vi "UIinit_Main.vi"(10 "VIref":refnum<vi>, 11 "Language":refnum<vi>) -> ()   [LabVIEW 2015]
uses:
  GlobalVar.vi
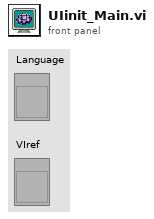
[diagram p1: front panel]
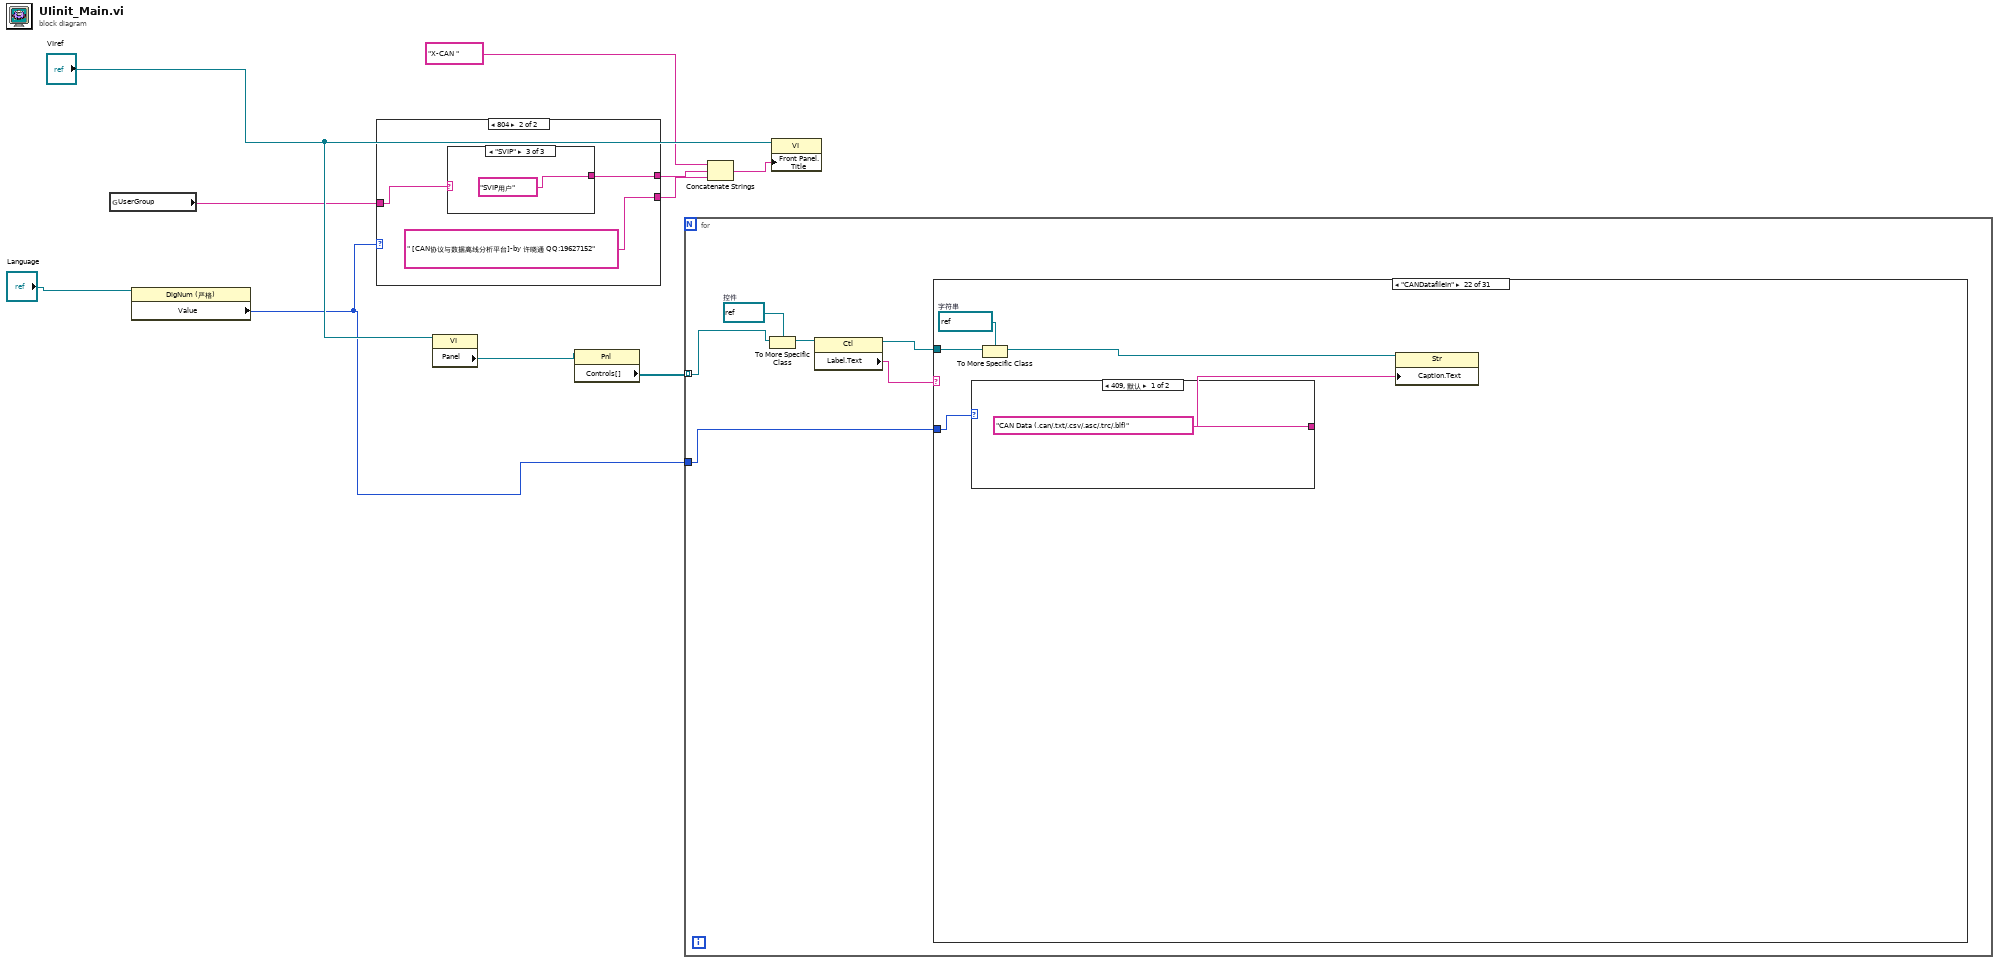
[diagram p0: block diagram]
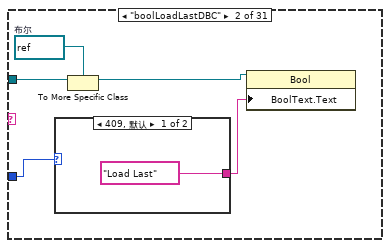
[diagram p3: hidden frame]
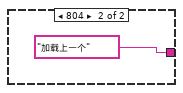
[diagram p4: hidden frame]
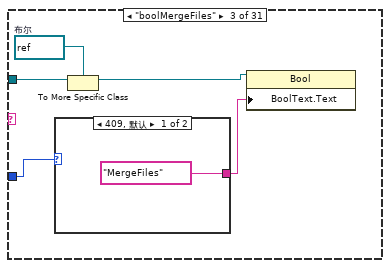
[diagram p5: hidden frame]
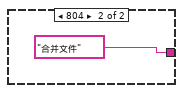
[diagram p6: hidden frame]
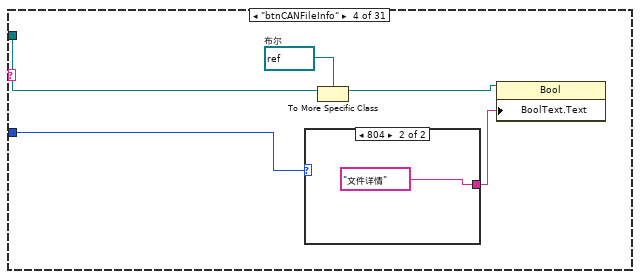
[diagram p7: hidden frame]
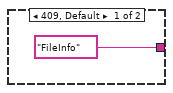
[diagram p8: hidden frame]
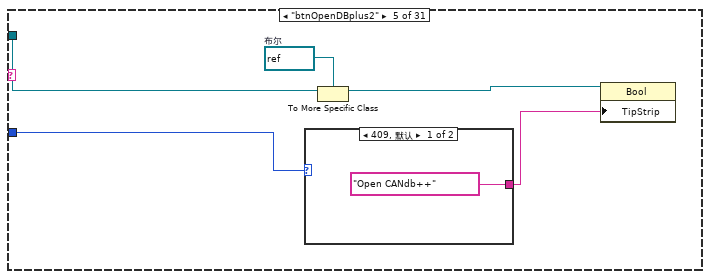
[diagram p9: hidden frame]
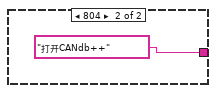
[diagram p10: hidden frame]
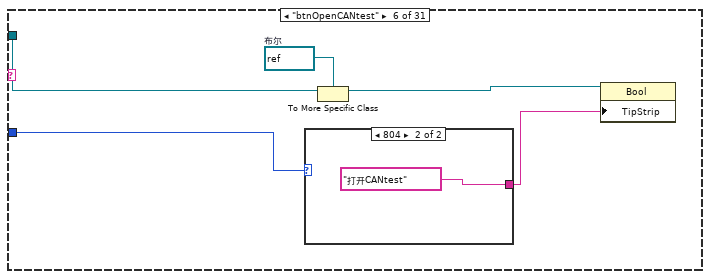
[diagram p11: hidden frame]
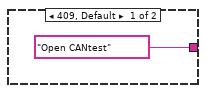
[diagram p12: hidden frame]
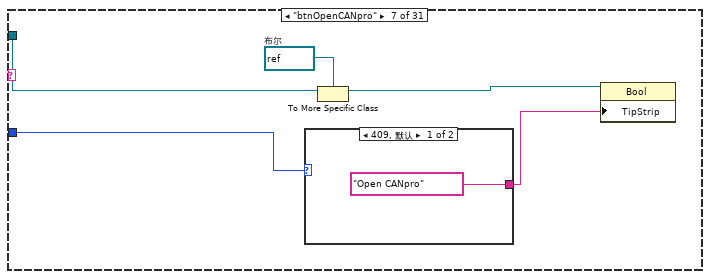
[diagram p13: hidden frame]
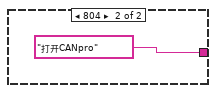
[diagram p14: hidden frame]
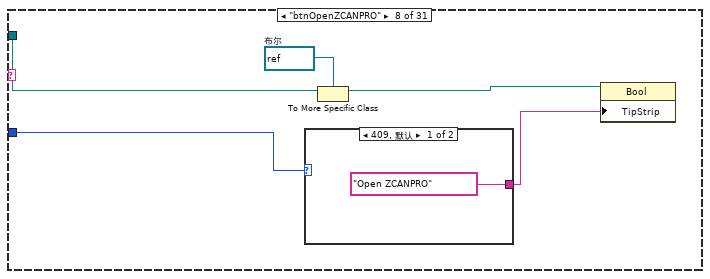
[diagram p15: hidden frame]
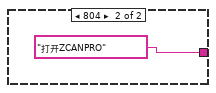
[diagram p16: hidden frame]
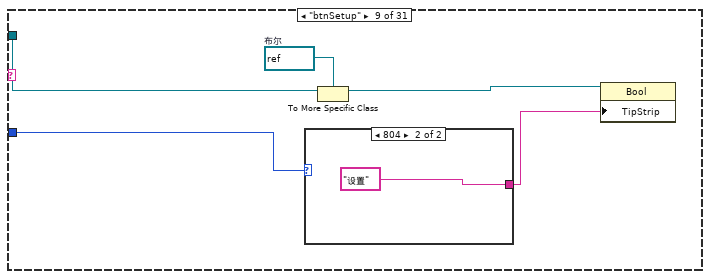
[diagram p17: hidden frame]
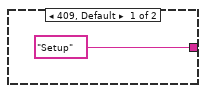
[diagram p18: hidden frame]
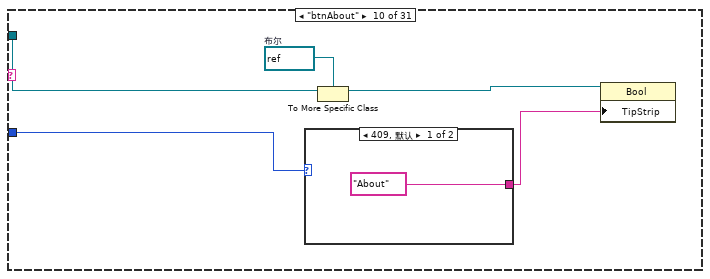
[diagram p19: hidden frame]
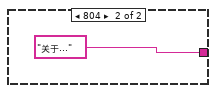
[diagram p20: hidden frame]
diagram:
  n1 = global read "GlobalVar.vi" "UserGroup"() -> (w2:string)
  n2 = property class="DigNum (严格)"(reference="Language") -> ("Value"=w6:u32)  [unwired: 1 in, 2 out]
  n3 = case shown="804" w6 {
    tunnel: [w12 " [CAN协议与数据离线分析平台]-by 许晓通 QQ:19627152"] -> w5
    tunnel: [w11 w13] -> w4
    tunnel: w2 -> [w11 w14]
    frame 409, Default {
      w12 = " [CAN Offline Analysis Platform]-by Jay Sur E-mail:jaysur@foxmail.com"  # [CAN Offline Analysis Platform]-by Jay Sur E-mail:jaysur@foxmail.com
    }
    frame 804 {
      n4 = case shown="\"SVIP\"" w14 {
        tunnel: ["普通用户" "VIP用户" "SVIP用户"] -> w13
        frame "假", Default {
        }
        frame "VIP" {
        }
        frame "SVIP" {
        }
      }
    }
  }
  n5 = property class="VI"(reference="VIref") -> ("Panel"=w7:refnum<vi>)  [unwired: 1 in, 2 out]
  n6 = property class="Pnl"(reference=w7) -> ("Controls[]"=w8:refnum<vi>[])  [unwired: 1 in, 2 out]
  n7 = for {
    tunnel: w8 -> [w19] mode=indexing
    tunnel: w6 -> [w20]
    w24 = refnum<vi> refnum  # 控件
    n8 = To More Specific Class(target class=w24, reference=w19) -> (specific class reference=w23:refnum<vi>)  [unwired: 1 in, 1 out]
    n9 = property class="Ctl"(reference=w23) -> (reference out=w21:refnum<vi>, "Label.Text"=w22:string)  [unwired: 1 in, 1 out]
    n10 = case shown="\"CANDatafileIn\"" w22 {
      tunnel: w21 -> [_ w28 w35 w42 w49 w56 w63 w70 w77 w84 w91 w98 w105 w113 w123 w132 w139 w146 w153 w160 w167 w174 w181 w188 w195 w202 w209 w216 w223 w231 w287]
      tunnel: w20 -> [_ w29 w36 w43 w50 w57 w64 w71 w78 w85 w92 w99 w106 w114 w124 w133 w140 w147 w154 w161 w168 w175 w182 w189 w196 w203 w210 w217 w224 w227 w292]
      frame "假", Default {
      }
      frame "boolLoadLastDBC" {
        w27 = refnum<vi> refnum  # 布尔
        n11 = case shown="409, 默认" w29 {
          tunnel: ["Load Last" "加载上一个"] -> w25
          frame 409, Default {
          }
          frame 804 {
          }
        }
        n12 = To More Specific Class(target class=w27, reference=w28) -> (specific class reference=w26:refnum<vi>)  [unwired: 1 in, 1 out]
        n13 = property class="Bool"(reference=w26, "BoolText.Text"=w25) -> ()  [unwired: 1 in, 2 out]
      }
      frame "boolMergeFiles" {
        w34 = refnum<vi> refnum  # 布尔
        n14 = case shown="409, 默认" w36 {
          tunnel: ["MergeFiles" "合并文件"] -> w32
          frame 409, Default {
          }
          frame 804 {
          }
        }
        n15 = To More Specific Class(target class=w34, reference=w35) -> (specific class reference=w33:refnum<vi>)  [unwired: 1 in, 1 out]
        n16 = property class="Bool"(reference=w33, "BoolText.Text"=w32) -> ()  [unwired: 1 in, 2 out]
      }
      frame "btnCANFileInfo" {
        w41 = refnum<vi> refnum  # 布尔
        n17 = case shown="804" w43 {
          tunnel: ["FileInfo" "文件详情"] -> w39
          frame 409, Default {
          }
          frame 804 {
          }
        }
        n18 = To More Specific Class(target class=w41, reference=w42) -> (specific class reference=w40:refnum<vi>)  [unwired: 1 in, 1 out]
        n19 = property class="Bool"(reference=w40, "BoolText.Text"=w39) -> ()  [unwired: 1 in, 2 out]
      }
      frame "btnOpenDBplus2" {
        w48 = refnum<vi> refnum  # 布尔
        n20 = case shown="409, 默认" w50 {
          tunnel: ["Open CANdb++" "打开CANdb++"] -> w46
          frame 409, Default {
          }
          frame 804 {
          }
        }
        n21 = To More Specific Class(target class=w48, reference=w49) -> (specific class reference=w47:refnum<vi>)  [unwired: 1 in, 1 out]
        n22 = property class="Bool"(reference=w47, "TipStrip"=w46) -> ()  [unwired: 1 in, 2 out]
      }
      frame "btnOpenCANtest" {
        w55 = refnum<vi> refnum  # 布尔
        n23 = case shown="804" w57 {
          tunnel: ["Open CANtest" "打开CANtest"] -> w53
          frame 409, Default {
          }
          frame 804 {
          }
        }
        n24 = To More Specific Class(target class=w55, reference=w56) -> (specific class reference=w54:refnum<vi>)  [unwired: 1 in, 1 out]
        n25 = property class="Bool"(reference=w54, "TipStrip"=w53) -> ()  [unwired: 1 in, 2 out]
      }
      frame "btnOpenCANpro" {
        w62 = refnum<vi> refnum  # 布尔
        n26 = case shown="409, 默认" w64 {
          tunnel: ["Open CANpro" "打开CANpro"] -> w60
          frame 409, Default {
          }
          frame 804 {
          }
        }
        n27 = To More Specific Class(target class=w62, reference=w63) -> (specific class reference=w61:refnum<vi>)  [unwired: 1 in, 1 out]
        n28 = property class="Bool"(reference=w61, "TipStrip"=w60) -> ()  [unwired: 1 in, 2 out]
      }
      frame "btnOpenZCANPRO" {
        w69 = refnum<vi> refnum  # 布尔
        n29 = case shown="409, 默认" w71 {
          tunnel: ["Open ZCANPRO" "打开ZCANPRO"] -> w67
          frame 409, Default {
          }
          frame 804 {
          }
        }
        n30 = To More Specific Class(target class=w69, reference=w70) -> (specific class reference=w68:refnum<vi>)  [unwired: 1 in, 1 out]
        n31 = property class="Bool"(reference=w68, "TipStrip"=w67) -> ()  [unwired: 1 in, 2 out]
      }
      frame "btnSetup" {
        w76 = refnum<vi> refnum  # 布尔
        n32 = case shown="804" w78 {
          tunnel: ["Setup" "设置"] -> w74
          frame 409, Default {
          }
          frame 804 {
          }
        }
        n33 = To More Specific Class(target class=w76, reference=w77) -> (specific class reference=w75:refnum<vi>)  [unwired: 1 in, 1 out]
        n34 = property class="Bool"(reference=w75, "TipStrip"=w74) -> ()  [unwired: 1 in, 2 out]
      }
      frame "btnAbout" {
        w83 = refnum<vi> refnum  # 布尔
        n35 = case shown="409, 默认" w85 {
          tunnel: ["About" "关于..."] -> w81
          frame 409, Default {
          }
          frame 804 {
          }
        }
        n36 = To More Specific Class(target class=w83, reference=w84) -> (specific class reference=w82:refnum<vi>)  [unwired: 1 in, 1 out]
        n37 = property class="Bool"(reference=w82, "TipStrip"=w81) -> ()  [unwired: 1 in, 2 out]
      }
      frame "btnDonate" {
        w90 = refnum<vi> refnum  # 布尔
        n38 = case shown="804" w92 {
          tunnel: ["Donate" "捐赠"] -> w88
          frame 409, Default {
          }
          frame 804 {
          }
        }
        n39 = To More Specific Class(target class=w90, reference=w91) -> (specific class reference=w89:refnum<vi>)  [unwired: 1 in, 1 out]
        n40 = property class="Bool"(reference=w89, "TipStrip"=w88) -> ()  [unwired: 1 in, 2 out]
      }
      frame "btnUpdateChk" {
        w97 = refnum<vi> refnum  # 布尔
        n41 = case shown="409, 默认" w99 {
          tunnel: ["Check Upadte" "检查更新"] -> w95
          frame 409, Default {
          }
          frame 804 {
          }
        }
        n42 = To More Specific Class(target class=w97, reference=w98) -> (specific class reference=w96:refnum<vi>)  [unwired: 1 in, 1 out]
        n43 = property class="Bool"(reference=w96, "TipStrip"=w95) -> ()  [unwired: 1 in, 2 out]
      }
      frame "ClearSelectedSig" {
        w104 = refnum<vi> refnum  # 布尔
        n44 = case shown="409, 默认" w106 {
          tunnel: ["Empty" "清空"] -> w102
          frame 409, Default {
          }
          frame 804 {
          }
        }
        n45 = To More Specific Class(target class=w104, reference=w105) -> (specific class reference=w103:refnum<vi>)  [unwired: 1 in, 1 out]
        n46 = property class="Bool"(reference=w103, "BoolText.Text"=w102) -> ()  [unwired: 1 in, 2 out]
      }
      frame "LookAllSigDefinition" {
        w112 = refnum<vi> refnum  # 布尔
        n47 = To More Specific Class(target class=w112, reference=w113) -> (specific class reference=w110:refnum<vi>)  [unwired: 1 in, 1 out]
        n48 = case shown="804" w114 {
          tunnel: ["AllVal" "所有值表"] -> w111
          tunnel: ["Look values of all signals " "查看所有信号的值表"] -> w109
          frame 409, Default {
          }
          frame 804 {
          }
        }
        n49 = property class="Bool"(reference=w110, "BoolText.Text"=w111) -> ()  [unwired: 1 in, 2 out]
        n50 = property class="Bool"(reference=w110, "TipStrip"=w109) -> ()  [unwired: 1 in, 2 out]
      }
      frame "LookSelSigDefinition" {
        w122 = refnum<vi> refnum  # 布尔
        n51 = To More Specific Class(target class=w122, reference=w123) -> (specific class reference=w120:refnum<vi>)  [unwired: 1 in, 1 out]
        n52 = case shown="804" w124 {
          tunnel: ["SelVal" "已选值表"] -> w121
          tunnel: ["Look values of selected signals " "查看已选信号的值表"] -> w119
          frame 409, Default {
          }
          frame 804 {
          }
        }
        n53 = property class="Bool"(reference=w120, "BoolText.Text"=w121) -> ()  [unwired: 1 in, 2 out]
        n54 = property class="Bool"(reference=w120, "TipStrip"=w119) -> ()  [unwired: 1 in, 2 out]
      }
      frame "boolDrawGraph" {
        w131 = refnum<vi> refnum  # 布尔
        n55 = case shown="804" w133 {
          tunnel: ["Draw" "绘图"] -> w129
          frame 409, Default {
          }
          frame 804 {
          }
        }
        n56 = To More Specific Class(target class=w131, reference=w132) -> (specific class reference=w130:refnum<vi>)  [unwired: 1 in, 1 out]
        n57 = property class="Bool"(reference=w130, "BoolText.Text"=w129) -> ()  [unwired: 1 in, 2 out]
      }
      frame "ClearMainGraph" {
        w138 = refnum<vi> refnum  # 布尔
        n58 = case shown="409, 默认" w140 {
          tunnel: ["Clear" "清空主图"] -> w136
          frame 409, Default {
          }
          frame 804 {
          }
        }
        n59 = To More Specific Class(target class=w138, reference=w139) -> (specific class reference=w137:refnum<vi>)  [unwired: 1 in, 1 out]
        n60 = property class="Bool"(reference=w137, "BoolText.Text"=w136) -> ()  [unwired: 1 in, 2 out]
      }
      frame "boolExport2Excel" {
        w145 = refnum<vi> refnum  # 布尔
        n61 = case shown="804" w147 {
          tunnel: ["Export2Excel" "导出至Excel"] -> w143
          frame 409, Default {
          }
          frame 804 {
          }
        }
        n62 = To More Specific Class(target class=w145, reference=w146) -> (specific class reference=w144:refnum<vi>)  [unwired: 1 in, 1 out]
        n63 = property class="Bool"(reference=w144, "BoolText.Text"=w143) -> ()  [unwired: 1 in, 2 out]
      }
      frame "DBCpath" {
        w152 = refnum<vi> refnum  # 路径
        n64 = case shown="409, 默认" w154 {
          tunnel: ["DBC File (.dbc)" "DBC文件（.dbc）"] -> w150
          frame 409, Default {
          }
          frame 804 {
          }
        }
        n65 = To More Specific Class(target class=w152, reference=w153) -> (specific class reference=w151:refnum<vi>)  [unwired: 1 in, 1 out]
        n66 = property class="Path"(reference=w151, "Caption.Text"=w150) -> ()  [unwired: 1 in, 2 out]
      }
      frame "DBCfileIn" {
        w159 = refnum<vi> refnum  # 字符串
        n67 = case shown="409, 默认" w161 {
          tunnel: ["DBC File (.dbc)" "DBC文件（.dbc）"] -> w157
          frame 409, Default {
          }
          frame 804 {
          }
        }
        n68 = To More Specific Class(target class=w159, reference=w160) -> (specific class reference=w158:refnum<vi>)  [unwired: 1 in, 1 out]
        n69 = property class="Str"(reference=w158, "Caption.Text"=w157) -> ()  [unwired: 1 in, 2 out]
      }
      frame "CANpath" {
        w166 = refnum<vi> refnum  # 路径
        n70 = case shown="804" w168 {
          tunnel: ["CAN Data (.can/.txt/.csv/.asc/.trc)" "CAN离线数据（.can/.txt/.csv/.asc/.trc）"] -> w164
          frame 409, Default {
          }
          frame 804 {
          }
        }
        n71 = To More Specific Class(target class=w166, reference=w167) -> (specific class reference=w165:refnum<vi>)  [unwired: 1 in, 1 out]
        n72 = property class="Path"(reference=w165, "Caption.Text"=w164) -> ()  [unwired: 1 in, 2 out]
      }
      frame "CANDatafileIn" {
        w173 = refnum<vi> refnum  # 字符串
        n73 = case shown="409, 默认" w175 {
          tunnel: ["CAN Data (.can/.txt/.csv/.asc/.trc/.blf)" "CAN离线数据（.can/.txt/.csv/.asc/.trc/.blf）"] -> w171
          frame 409, Default {
          }
          frame 804 {
          }
        }
        n74 = To More Specific Class(target class=w173, reference=w174) -> (specific class reference=w172:refnum<vi>)  [unwired: 1 in, 1 out]
        n75 = property class="Str"(reference=w172, "Caption.Text"=w171) -> ()  [unwired: 1 in, 2 out]
      }
      frame "CANmessageNum" {
        w180 = refnum<vi> refnum  # 数值
        n76 = case shown="409, 默认" w182 {
          tunnel: ["Msg" "报文数"] -> w178
          frame 409, Default {
          }
          frame 804 {
          }
        }
        n77 = To More Specific Class(target class=w180, reference=w181) -> (specific class reference=w179:refnum<vi>)  [unwired: 1 in, 1 out]
        n78 = property class="Num"(reference=w179, "Caption.Text"=w178) -> ()  [unwired: 1 in, 2 out]
      }
      frame "SigNum" {
        w187 = refnum<vi> refnum  # 数值
        n79 = case shown="409, 默认" w189 {
          tunnel: ["Sig" "信号数"] -> w185
          frame 409, Default {
          }
          frame 804 {
          }
        }
        n80 = To More Specific Class(target class=w187, reference=w188) -> (specific class reference=w186:refnum<vi>)  [unwired: 1 in, 1 out]
        n81 = property class="Num"(reference=w186, "Caption.Text"=w185) -> ()  [unwired: 1 in, 2 out]
      }
      frame "CanMessageRowsNum" {
        w194 = refnum<vi> refnum  # 数值
        n82 = case shown="409, 默认" w196 {
          tunnel: ["Rows" "报文数"] -> w192
          frame 409, Default {
          }
          frame 804 {
          }
        }
        n83 = To More Specific Class(target class=w194, reference=w195) -> (specific class reference=w193:refnum<vi>)  [unwired: 1 in, 1 out]
        n84 = property class="Num"(reference=w193, "Caption.Text"=w192) -> ()  [unwired: 1 in, 2 out]
      }
      frame "NumSelected" {
        w201 = refnum<vi> refnum  # 数值
        n85 = case shown="409, 默认" w203 {
          tunnel: ["Selected" "已选数量"] -> w199
          frame 409, Default {
          }
          frame 804 {
          }
        }
        n86 = To More Specific Class(target class=w201, reference=w202) -> (specific class reference=w200:refnum<vi>)  [unwired: 1 in, 1 out]
        n87 = property class="Num"(reference=w200, "Caption.Text"=w199) -> ()  [unwired: 1 in, 2 out]
      }
      frame "MainGraph" {
        w208 = refnum<vi> refnum  # XY图
        n88 = case shown="409, 默认" w210 {
          tunnel: ["Time/s" "时间/s"] -> w206
          frame 409, Default {
          }
          frame 804 {
          }
        }
        n89 = To More Specific Class(target class=w208, reference=w209) -> (specific class reference=w207:refnum<vi>)  [unwired: 1 in, 1 out]
        n90 = property class="XYGraph"(reference=w207, "XScale.NameLbl.Text"=w206) -> ()  [unwired: 1 in, 2 out]
      }
      frame "ListOfDBC" {
        w215 = refnum<vi> refnum  # 树形控件
        n91 = case shown="409, 默认" w217 {
          tunnel: [string[] ["Msg&Sig", "StartB", "Len", "ByteOd", "Factor", "Offset", "Min", "Max", "Unit", "Node", "Sign"] string[] ["报文及信号", "起始位", "长度", "格式", "缩放系数", "偏移量", "最小值", "最大值", "单位", "节点", "符号"]] -> w213
          frame 409, Default {
          }
          frame 804 {
          }
        }
        n92 = To More Specific Class(target class=w215, reference=w216) -> (specific class reference=w214:refnum<vi>)  [unwired: 1 in, 1 out]
        n93 = property class="Tree"(reference=w214, "ColHdrString"=w213) -> ()  [unwired: 1 in, 2 out]
      }
      frame "SelectedSigList" {
        w222 = refnum<vi> refnum  # 多列列表框
        n94 = case shown="409, 默认" w224 {
          tunnel: [string[] ["Signal", "Unit"] string[] ["信号", "单位"]] -> w220
          frame 409, Default {
          }
          frame 804 {
          }
        }
        n95 = To More Specific Class(target class=w222, reference=w223) -> (specific class reference=w221:refnum<vi>)  [unwired: 1 in, 1 out]
        n96 = property class="MCListbox"(reference=w221, "ColHdrString"=w220) -> ()  [unwired: 1 in, 2 out]
      }
      frame "AxleConfigTabs" {
        w230 = refnum<vi> refnum  # 选项卡控件
        n97 = To More Specific Class(target class=w230, reference=w231) -> (specific class reference=w229:refnum<vi>)  [unwired: 1 in, 1 out]
        n98 = property class="TabCtl"(reference=w229) -> ("Pages"=w228:refnum<vi>[])  [unwired: 1 in, 2 out]
        n99 = for {
          tunnel: w228 -> [w235] mode=indexing
          tunnel: w227 -> [w232]
          w236 = refnum<vi> refnum  # 选项卡
          n100 = To More Specific Class(target class=w236, reference=w235) -> (specific class reference=w233:refnum<vi>)  [unwired: 1 in, 1 out]
          n101 = property class="Page"(reference=w233) -> ("ControlsOnPage"=w234:refnum<vi>[])  [unwired: 1 in, 2 out]
          n102 = for {
            tunnel: w234 -> [w239] mode=indexing
            tunnel: w232 -> [w240]
            w244 = refnum<vi> refnum  # 控件
            n103 = To More Specific Class(target class=w244, reference=w239) -> (specific class reference=w243:refnum<vi>)  [unwired: 1 in, 1 out]
            n104 = property class="Ctl"(reference=w243) -> (reference out=w241:refnum<vi>, "Label.Text"=w242:string)  [unwired: 1 in, 1 out]
            n105 = case shown="\"TimeFormat\"" w242 {
              tunnel: w241 -> [_ w248 w255 w262 w271]
              tunnel: w240 -> [_ w249 w256 w263 w270]
              frame "假", Default {
              }
              frame "btnConfigYandCurves" {
                w247 = refnum<vi> refnum  # 布尔
                n106 = case shown="804" w249 {
                  tunnel: ["ConfigY&Lines" "配置Y轴和定义曲线名"] -> w245
                  frame 409, Default {
                  }
                  frame 804 {
                  }
                }
                n107 = To More Specific Class(target class=w247, reference=w248) -> (specific class reference=w246:refnum<vi>)  [unwired: 1 in, 1 out]
                n108 = property class="Bool"(reference=w246, "BoolText.Text"=w245) -> ()  [unwired: 1 in, 2 out]
              }
              frame "isAutoY" {
                w254 = refnum<vi> refnum  # 布尔
                n109 = case shown="409, 默认" w256 {
                  tunnel: ["AutoY" "自动Y轴"] -> w252
                  frame 409, Default {
                  }
                  frame 804 {
                  }
                }
                n110 = To More Specific Class(target class=w254, reference=w255) -> (specific class reference=w253:refnum<vi>)  [unwired: 1 in, 1 out]
                n111 = property class="Bool"(reference=w253, "Caption.Text"=w252) -> ()  [unwired: 1 in, 2 out]
              }
              frame "isAutoCurves" {
                w261 = refnum<vi> refnum  # 布尔
                n112 = case shown="804" w263 {
                  tunnel: ["AutoLine" "自动配线"] -> w259
                  frame 409, Default {
                  }
                  frame 804 {
                  }
                }
                n113 = To More Specific Class(target class=w261, reference=w262) -> (specific class reference=w260:refnum<vi>)  [unwired: 1 in, 1 out]
                n114 = property class="Bool"(reference=w260, "Caption.Text"=w259) -> ()  [unwired: 1 in, 2 out]
              }
              frame "TimeFormat" {
                w272 = refnum<vi> refnum  # 下拉列表
                n115 = case shown="804" w270 {
                  tunnel: [string[] ["Relative(s)", "Abs(noDate)", "Abs(withDate)"] string[] ["相对时间(秒)", "绝对时间(无日期)", "绝对时间(带日期)"]] -> w269
                  tunnel: ["TimeFormat" "时间轴格式"] -> w266
                  frame 409, Default {
                  }
                  frame 804 {
                  }
                }
                n116 = To More Specific Class(target class=w272, reference=w271) -> (specific class reference=w268:refnum<vi>)  [unwired: 1 in, 1 out]
                n117 = property class="Ring"(reference=w268, "Caption.Text"=w266) -> (reference out=w267:refnum<vi>)  [unwired: 1 in, 1 out]
                n118 = property class="Ring"(reference=w267, "Strings []"=w269) -> ()  [unwired: 1 in, 2 out]
              }
            }
          }
          n119 = property class="Page"(reference=w233) -> (reference out=w237:refnum<vi>, "PageLabel"=w238:string)  [unwired: 1 in, 1 out]
          n120 = case shown="\"Yset\"" w238 {
            tunnel: w232 -> [_ w279 w284]
            tunnel: w237 -> [_ w278 w283]
            frame "假", Default {
            }
            frame "Xset" {
              n121 = case shown="409, 默认" w279 {
                tunnel: ["X axis" "X轴"] -> w277
                frame 409, Default {
                }
                frame 804 {
                }
              }
              n122 = property class="Page"(reference=w278, "TabCaption"=w277) -> ()  [unwired: 1 in, 2 out]
            }
            frame "Yset" {
              n123 = case shown="804" w284 {
                tunnel: ["Y axis" "Y轴"] -> w282
                frame 409, Default {
                }
                frame 804 {
                }
              }
              n124 = property class="Page"(reference=w283, "TabCaption"=w282) -> ()  [unwired: 1 in, 2 out]
            }
          }
        }
      }
      frame "btnConfigYandCurves" {
        w291 = refnum<vi> refnum  # 控件
        n125 = To More Specific Class(target class=w291, reference=w287) -> (specific class reference=w290:refnum<vi>)  [unwired: 1 in, 1 out]
        n126 = property class="Ctl"(reference=w290) -> (reference out=w288:refnum<vi>, "Label.Text"=w289:string)  [unwired: 1 in, 1 out]
        n127 = case shown="\"btnConfigYandCurves\"" w289 {
          tunnel: w288 -> [_ w296 w303 w310 w319]
          tunnel: w292 -> [_ w297 w304 w311 w318]
          frame "假", Default {
          }
          frame "btnConfigYandCurves" {
            w295 = refnum<vi> refnum  # 布尔
            n128 = case shown="409, 默认" w297 {
              tunnel: ["ConfigY&Lines" "配置Y轴和曲线名"] -> w293
              frame 409, Default {
              }
              frame 804 {
              }
            }
            n129 = To More Specific Class(target class=w295, reference=w296) -> (specific class reference=w294:refnum<vi>)  [unwired: 1 in, 1 out]
            n130 = property class="Bool"(reference=w294, "BoolText.Text"=w293) -> ()  [unwired: 1 in, 2 out]
          }
          frame "isAutoY" {
            w302 = refnum<vi> refnum  # 布尔
            n131 = case shown="409, 默认" w304 {
              tunnel: ["AutoY" "自动Y轴"] -> w300
              frame 409, Default {
              }
              frame 804 {
              }
            }
            n132 = To More Specific Class(target class=w302, reference=w303) -> (specific class reference=w301:refnum<vi>)  [unwired: 1 in, 1 out]
            n133 = property class="Bool"(reference=w301, "Caption.Text"=w300) -> ()  [unwired: 1 in, 2 out]
          }
          frame "isAutoCurves" {
            w309 = refnum<vi> refnum  # 布尔
            n134 = case shown="804" w311 {
              tunnel: ["AutoLine" "自动配线"] -> w307
              frame 409, Default {
              }
              frame 804 {
              }
            }
            n135 = To More Specific Class(target class=w309, reference=w310) -> (specific class reference=w308:refnum<vi>)  [unwired: 1 in, 1 out]
            n136 = property class="Bool"(reference=w308, "Caption.Text"=w307) -> ()  [unwired: 1 in, 2 out]
          }
          frame "TimeFormat" {
            w320 = refnum<vi> refnum  # 下拉列表
            n137 = case shown="804" w318 {
              tunnel: [string[] ["Relative(s)", "Abs(noDate)", "Abs(withDate)"] string[] ["相对时间(秒)", "绝对时间(无日期)", "绝对时间(带日期)"]] -> w317
              tunnel: ["TimeFormat" "时间轴格式"] -> w314
              frame 409, Default {
              }
              frame 804 {
              }
            }
            n138 = To More Specific Class(target class=w320, reference=w319) -> (specific class reference=w316:refnum<vi>)  [unwired: 1 in, 1 out]
            n139 = property class="Ring"(reference=w316, "Caption.Text"=w314) -> (reference out=w315:refnum<vi>)  [unwired: 1 in, 1 out]
            n140 = property class="Ring"(reference=w315, "Strings []"=w317) -> ()  [unwired: 1 in, 2 out]
          }
        }
      }
    }
  }
  n141 = Concatenate Strings("X-CAN ", w4, w5) -> (w1:string)
  n142 = property class="VI"(reference="VIref", "Front Panel.Title"=w1) -> ()  [unwired: 1 in, 2 out]
